vi "Tegam4040 - Low Pass Filter.vi"(0 "Instrument Session Handle In":u32 format="%x", 1 "LP Filter":enum16{"No Filter", "100kHz", "1MHz"}(ring), 11 "error in (no error)":errorcluster) -> (4 "Instrument Session Handle Out (dupl)":u32 format="%x", 15 "error out":errorcluster)   [LabVIEW 2010, in "Tegam4040.lvlib"]
doc: "Low Pass Filter: Bits 9-10.\n\n0: No Filtering\n1: 100kHz Filter\n2: 1MHz Filter\n\n\nCalibration bit will be reset if attuation is changed."
uses:
  Tegam4040.lvlib
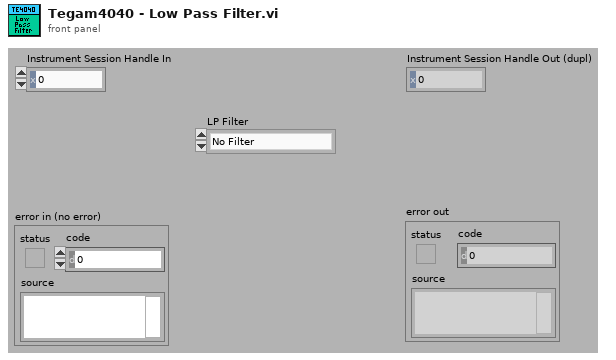
[diagram p1: front panel]
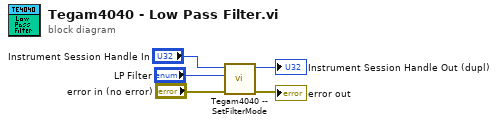
[diagram p0: block diagram]
diagram:
  n1 = call "Tegam4040 -- SetFilterMode.vi"("error in (no error)"="error in (no error)", "LP Filter"="LP Filter", "Instrument Session Handle In"="Instrument Session Handle In") -> ("error out"=→"error out":errorcluster, "Instrument Session Handle Out (dupl)"=→"Instrument Session Handle Out (dupl)":u32)  [unwired: 7 in]
